vi "calc_rjx_scale.vi"(11 "R+jX_Norm":cluster{"R":dbl, "jX":dbl}) -> (3 "R+jX_Scale":cluster{"R":dbl, "jX":dbl})   [LabVIEW 2025]
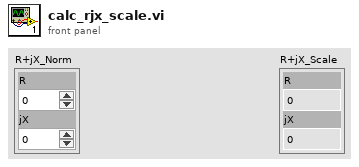
[diagram p1: front panel]
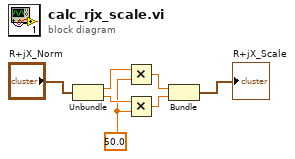
[diagram p0: block diagram]
diagram:
  w5 = 50.0 ("y")
  n1 = Unbundle("R+jX_Norm") -> ("R"=w7:dbl, "jX"=w6:dbl)
  n2 = Multiply(x=w7, y=w5) -> (x*y=w4:dbl)
  n3 = Multiply(x=w6, y=w5) -> (x*y=w3:dbl)
  n4 = Bundle(w4, w3) -> (→"R+jX_Scale":cluster{dbl, dbl})  [unwired: 1 in]
